vi "readFromXML.vi"(8 "error in (no error)":errorcluster, 10 "XML in":string, 11 "AmLimit in":refnum<class "AmLimit.lvclass">) -> (0 "error out":errorcluster, 3 "AmLimit out":refnum<class "AmLimit.lvclass">)   [LabVIEW 2022 SP3, in "TCSDataDefinitions.lvlib" / "TCSCommand.lvlib" / "AmLimit.lvclass"]
uses:
  AmLimit.lvclass
  AmLimit.lvclass/AmLimit.ctl
  TCSTcsCommand/TCSTcsCommand.lvclass
  <userlib>/Common/XML/XMLParser/XMLParser.lvclass
panel:
  out "airmass":dbl
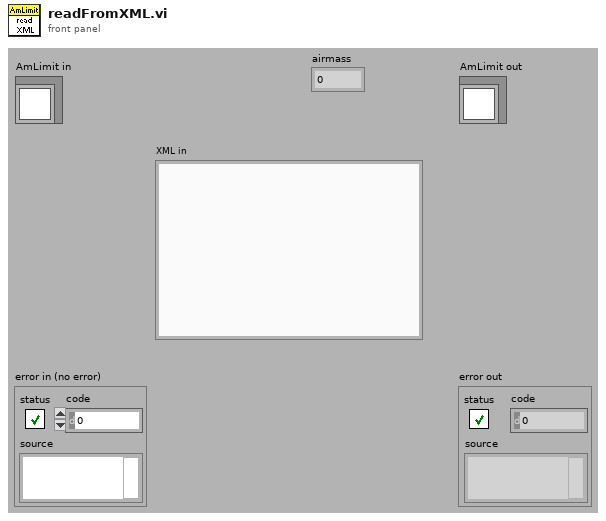
[diagram p1: front panel]
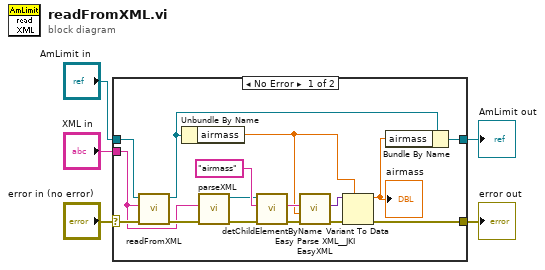
[diagram p0: block diagram]
diagram:
  n1 = case shown="No Error" "error in (no error)" {
    selector: "error in (no error)" -> [w16 w23]
    tunnel: [w9 w23] -> w4
    tunnel: [w19 w22] -> w2
    tunnel: "AmLimit in" -> [w18 w22]
    tunnel: "XML in" -> [w14 _]
    frame No Error {
      n2 = call-parent "readFromXML.vi"("error in (no error)"=w16, "XMLin"=w14, "TCSTcsCommand in"=w18) -> ("error out"=w15:errorcluster, "TCSTcsCommand out"=w17:refnum<class "AmLimit.lvclass">)  [unwired: 7 out]
      n3 = Unbundle By Name(w17) -> ("airmass"=w8:dbl)
      n4 = call <userlib>:"parseXML.vi"("error in (no error)"=w15, "XMLString in"=w14) -> ("error out"=w21:errorcluster, "Element out"=w6:refnum<class "XMLParser.lvclass">)  [unwired: 8 in]
      n5 = call <userlib>:"detChildElementByName.vi"("error in (no error)"=w21, "childName"="airmass" ("ChildName"), "Element in"=w6) -> ("error out"=w10:errorcluster, "childXML"=w11:string)  [unwired: 5 in, 2 out]
      n6 = call <vilib>:"Easy Parse XML__JKI EasyXML.vi"("error in (no error)"=w10, "LabVIEW Data (Type)"=w8, "XML String"=w11) -> ("error out"=w13:errorcluster, "LabVIEW Data"=w12:variant)  [unwired: 7 in]
      n7 = Variant To Data(error in=w13, type=w8, Variant=w12) -> (data=w7:dbl, error out=w9:errorcluster)
      "airmass" <- w7
      n8 = Bundle By Name(cluster=w17, "airmass"=w7) -> (w19:refnum<class "AmLimit.lvclass">)
    }
    frame Error {
    }
  }
  "error out" <- w4
  "AmLimit out" <- w2
